vi "Clock Cross Create Resources.vi"() -> (4 "resources":T1)   [LabVIEW 2020]
doc: "Creates resources for the register bus clock crossing VIs.\n\n<B>Output Parameters</B>\n\n<B>resources</B> contains references to the clock crossing FIFOs."
uses:
  Clock Cross Resources.ctl
  <vilib>/rvi/DataTransferAndStorage/Container/Common/niFpgaContainerGetUniqueNameForEmu.vi
  <vilib>/rvi/DataTransferAndStorage/Container/Common/niFpgaContainerSetEmuInfo.vi
  <vilib>/rvi/eio/common/nirviEmuReportErrorAndStop.vi
  <vilib>/rvi/LocalResourceManager/LocalResourceManager.xnode
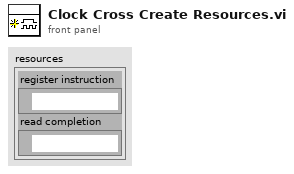
[diagram p1: front panel]
types:
  T1 = typedef "Clock Cross Resources.ctl" = cluster{"register instruction":refnum<k21>, "read completion":refnum<k21>}
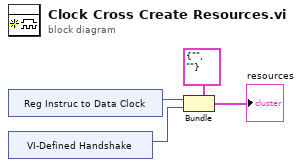
[diagram p0: block diagram]
diagram:
  n1 = xnode ("Reg Instruc to Data Clock")() -> ("FIFO Out"=w2:refnum<k21>)
  n2 = xnode "VI-Defined Handshake"() -> ("Handshake Out"=w1:refnum<k21>)
  n3 = Bundle(cluster=T1 {"register instruction"="", "read completion"=""} ("output cluster"), "register instruction"=w2, "read completion"=w1) -> (→"resources":T1)
